vi "Multi-Carrier Modulation.vi"() -> ()   [LabVIEW 2018]
uses:
  <vilib>/measure/maspectr.llb/FFT Spectrum (Real-Im) for 1 Chan.vi
  <vilib>/measure/NI_MAPro.lvlib
  <vilib>/addons/Modulation/niDMT.lvlib
panel:
  in  "Symbol Rate":i32=1
  out "Constellation Graph":T1(graph)
  in  "Carrier Method":T2(ring)
  out "FFT Complex":cluster{"f0":dbl, "df":dbl, "real part":dbl[]}(graph)
  out "FFT Real":cluster{"f0":dbl, "df":dbl, "real part":dbl[]}(graph)
  in  "QAM Comparison":enum16{"MT Modulate", "Homebrew"}(ring)
  out "Waveform Chart":dbl[](graph)
  out "Minimum Sampling Rate":dbl
  in  "Lowest f":dbl=1.0 format="%0.2p"
  in  "DataLen":i32=512
  in  "QAM Complexity":T3(ring)
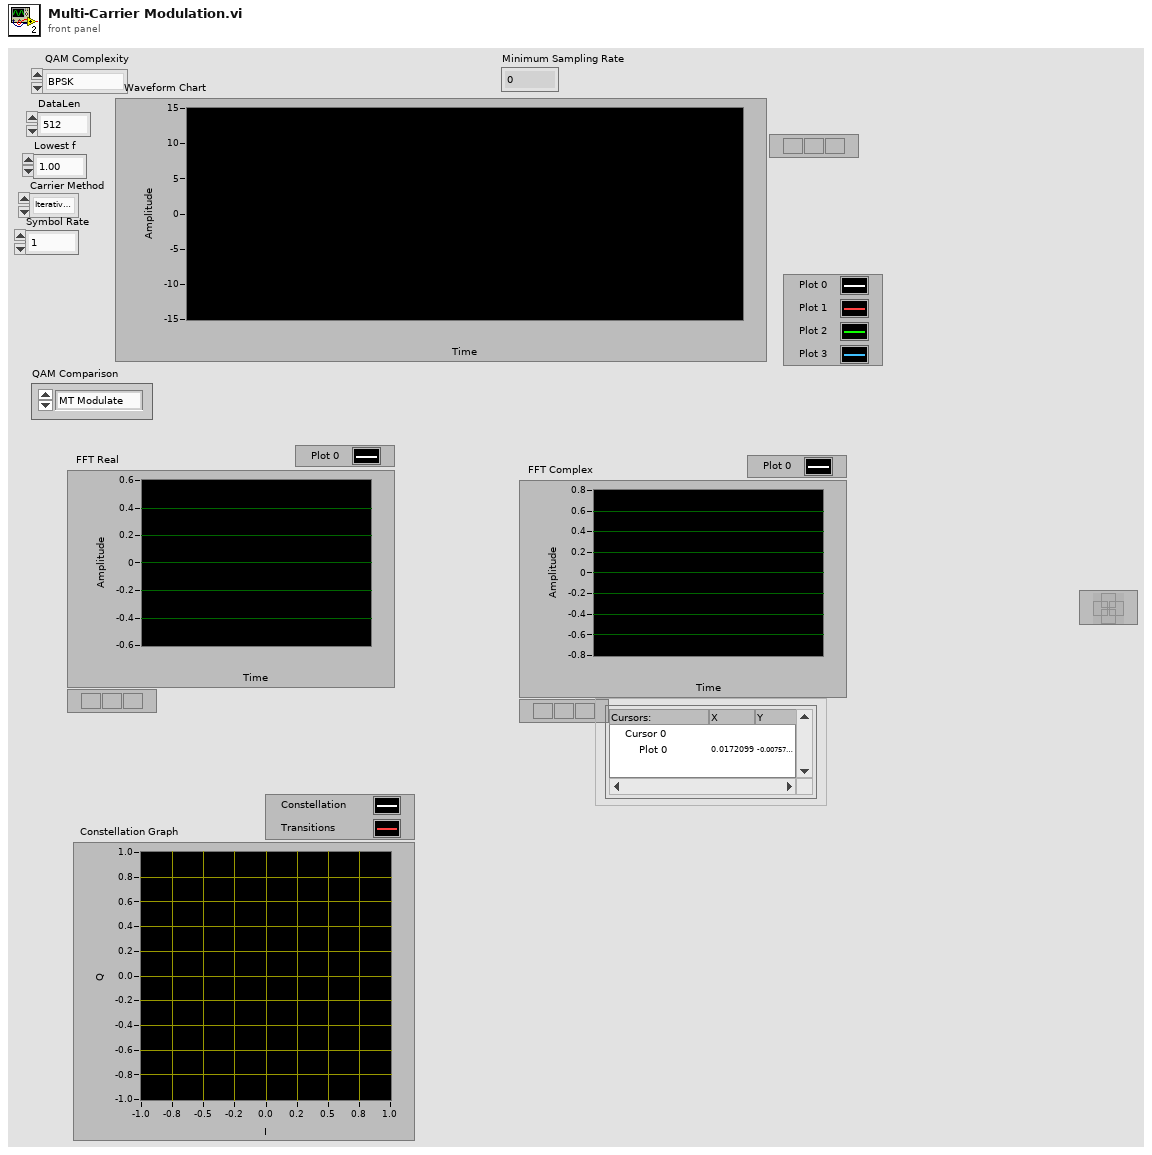
[diagram p1: front panel]
types:
  T1 = cluster{"Decimated Array":dbl[], "Decimated Array":dbl[]}[]
  T2 = enum16{"Iterative (Non-Reentrant)", "Crafted (Reentrant)"}
  T3 = enum16{"BPSK", "QPSK", "16-QAM", "64-QAM", "256-QAM"}
  T4 = typedef "NI_Matrix.lvlib/ComplexMatrix.ctl" = cdb[][]
  T5 = cluster{"f0":dbl, "df":dbl, "imaginary part":dbl[]}
  T6 = typedef "niAMT.lvlib/Complex Data Waveform.ctl" = cluster{"t0":dbl, "dt":dbl, "Y":cdb[]}
  T7 = cluster{"constellation":dbl[], "oversampled data":dbl[]}[]
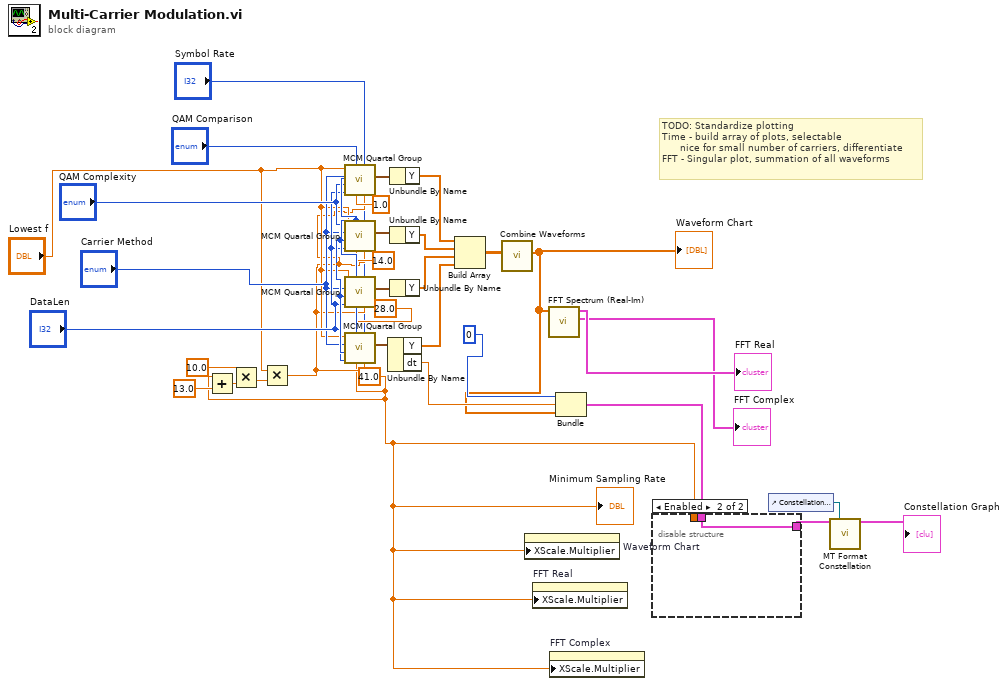
[diagram p0: block diagram]
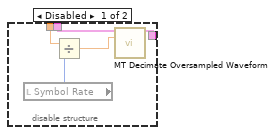
[diagram p2: hidden frame]
diagram:
  w6 = 41.0 ("y")
  # "TODO: Standardize plotting\nTime - build array of plots, selectable\n      nice for small number of carriers, differentiate\nFFT - Singular plot, summation of all waveforms"
  n1 = Add(x=w6, y=13.0) -> (x+y=w14:dbl)
  n2 = Multiply(x=10.0, y=w14) -> (x*y=w12:dbl)
  n3 = Multiply(x="Lowest f", y=w12) -> (x*y=w10:dbl)
  n4 = call "MCM Quartal Group.vi"("Sampling Rate"=w10, "Symbol Rate"="Symbol Rate", "Starting Subcarrier"=1.0 ("y"), "QAM Comparison"="QAM Comparison", "DataLen"="DataLen", "QAM Complexity"="QAM Complexity", "Carrier Method"="Carrier Method", "Lowest f"="Lowest f") -> ("output waveform"=w30:waveform(cdb))  [unwired: 3 out]
  n5 = call "MCM Quartal Group.vi"("Sampling Rate"=w10, "Symbol Rate"="Symbol Rate", "Starting Subcarrier"=14.0 ("y"), "QAM Comparison"="QAM Comparison", "DataLen"="DataLen", "QAM Complexity"="QAM Complexity", "Carrier Method"="Carrier Method", "Lowest f"="Lowest f") -> ("output waveform"=w29:waveform(cdb))  [unwired: 3 out]
  n6 = call "MCM Quartal Group.vi"("Sampling Rate"=w10, "Symbol Rate"="Symbol Rate", "Starting Subcarrier"=28.0 ("y"), "QAM Comparison"="QAM Comparison", "DataLen"="DataLen", "QAM Complexity"="QAM Complexity", "Carrier Method"="Carrier Method", "Lowest f"="Lowest f") -> ("output waveform"=w28:waveform(cdb))  [unwired: 3 out]
  n7 = call "MCM Quartal Group.vi"("Sampling Rate"=w10, "Symbol Rate"="Symbol Rate", "Starting Subcarrier"=w6, "QAM Comparison"="QAM Comparison", "DataLen"="DataLen", "QAM Complexity"="QAM Complexity", "Carrier Method"="Carrier Method", "Lowest f"="Lowest f") -> ("output waveform"=w27:waveform(cdb))  [unwired: 3 out]
  n8 = Unbundle By Name(w27) -> ("Y"=w23:cdb[], "dt"=w4:dbl)
  n9 = Unbundle By Name(w30) -> ("Y"=w26:cdb[])
  n10 = Unbundle By Name(w29) -> ("Y"=w25:cdb[])
  n11 = Unbundle By Name(w28) -> ("Y"=w24:cdb[])
  n12 = Build Array(w26, w25, w24, w23) -> (w22:T4)
  n13 = call "Combine Waveforms.vi"("Matrix of Carriers"=w22) -> ("Combined Output"=w3:cdb[])  [unwired: 10 in]
  "Waveform Chart" <- w3
  n14 = property on="Waveform Chart" class="WFChart (strict)"("XScale.Multiplier"=w6) -> ()  [unwired: 2 in, 2 out]
  n15 = property on="FFT Real" class="WFGraph (strict)"("XScale.Multiplier"=w6) -> ()  [unwired: 2 in, 2 out]
  n16 = call-poly <vilib>:"FFT Spectrum (Real-Im).vi"("time signal"=w3) -> ("imaginary part"=→"FFT Complex":T5, "real part"=→"FFT Real":cluster{"f0":dbl, "df":dbl, "real part":dbl[]})  [unwired: 6 in, 3 out]
  n17 = property on="FFT Complex" class="WFGraph (strict)"("XScale.Multiplier"=w6) -> ()  [unwired: 2 in, 2 out]
  n18 = Bundle(0, "dt"=w4, "Combined Output"=w3) -> (w2:cluster{i32, "dt":dbl, "Combined Output":cdb[]})  [unwired: 1 in]
  n19 = disable-structure shown="Enabled" {
    disable-tunnel: w6 -> [w38 _]
    disable-tunnel: w2 -> [w36 w39]
    disable-tunnel: [w35 w39] -> w1
    frame Disabled {
      n20 = local read "Symbol Rate"() -> (w37:i32)
      n21 = Divide(x=w38, y=w37) -> (x/y=w34:dbl)
      n22 = call <vilib>:"MT Decimate Oversampled Waveform.vi"("input complex waveform"=w36, "decimation factor"=w34) -> ("output complex waveform"=w35:T6)  [unwired: 12 in, 1 out]
    }
    frame Enabled {
    }
  }
  n23 = control-ref of="Constellation Graph"() -> (w9:refnum<vi>)
  n24 = call <vilib>:"MT Format Constellation.vi"("waveform"=w1, "constellation reference"=w9) -> ("constellation graph"=→"Constellation Graph":T7)  [unwired: 3 in, 10 out]
  "Minimum Sampling Rate" <- w6
